vi "main.vi"() -> ()   [LabVIEW 2019]
uses:
  System.Speech
panel:
  in  "Tab Control":T1(tab)
  out "B out 2":bool[][](array[boolean])
  out "A+B 4":bool[][](array[boolean])
  out "A out 2":bool[][](array[boolean])
  in  "A in 2":dbl
  in  "B in 2":dbl
  out "A+B 3":dbl
  out "NUMBER  2":string
  in  "A in":dbl
  in  "B in":dbl
  out "A+B 2":dbl
  out "B out":bool[](array[boolean])
  out "A out":bool[](array[boolean])
  out "A+B":bool[][](array[boolean])
  out "NUMBER":string
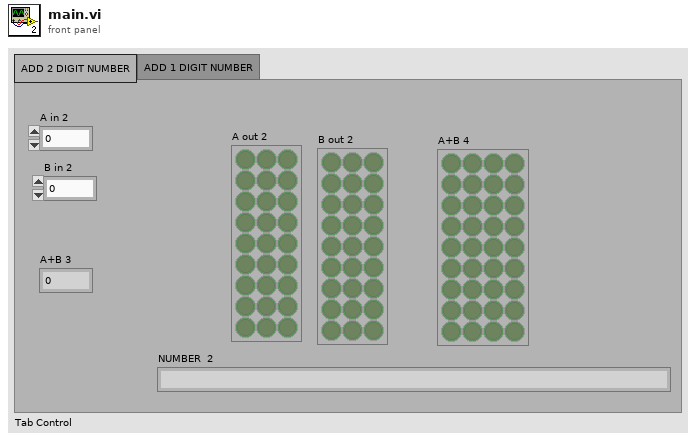
[diagram p1: front panel]
types:
  T1 = enum32{"ADD 2 DIGIT NUMBER", "ADD 1 DIGIT NUMBER"}
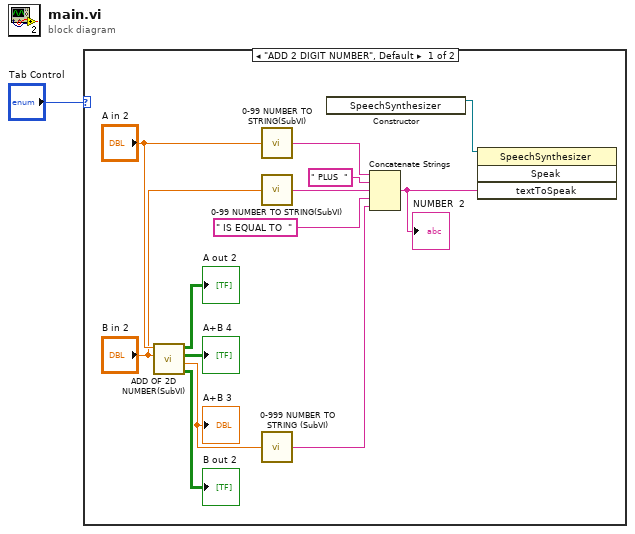
[diagram p0: block diagram]
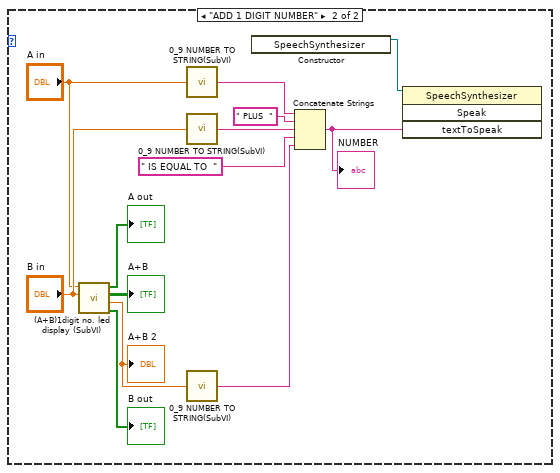
[diagram p2: hidden frame]
diagram:
  n1 = case shown="\"ADD 2 DIGIT NUMBER\", Default" "Tab Control" {
    frame "ADD 2 DIGIT NUMBER", Default {
      n2 = call "ADD OF 2D NUMBER(SubVI).vi"("B in"="B in 2", "A in"="A in 2") -> ("B out"=→"B out 2":bool[][], "A+B 2"=w2:dbl, "A+B"=→"A+B 4":bool[][], "A out"=→"A out 2":bool[][])  [unwired: 2 in]
      "A+B 3" <- w2
      n3 = call "0-99 NUMBER TO STRING(SubVI).vi"("A"="A in 2") -> ("element"=w9:string)
      n4 = call "0-99 NUMBER TO STRING(SubVI).vi"("A"="B in 2") -> ("element"=w7:string)
      n5 = call "0-999 NUMBER TO STRING (SubVI).vi"("A"=w2) -> ("element"=w3:string)
      n6 = constructor class="SpeechSynthesizer"() -> (reference out=w5:refnum<k24>)  [unwired: 3 in, 2 out]
      n7 = Concatenate Strings(w9, " PLUS  ", w7, " IS EQUAL TO  ", w3) -> (w4:string)
      "NUMBER  2" <- w4
      n8 = invoke class="SpeechSynthesizer" method="Speak"(reference=w5, "textToSpeak"=w4) -> ()  [unwired: 2 in, 4 out]
    }
    frame "ADD 1 DIGIT NUMBER" {
      n9 = call "(A+B)1digit no. led display (SubVI).vi"("B in"="B in", "A in"="A in") -> ("B out"=→"B out":bool[], "A+B 2"=w18:dbl, "A+B"=→"A+B":bool[][], "A out"=→"A out":bool[])  [unwired: 2 in]
      "A+B 2" <- w18
      n10 = call "0_9 NUMBER TO STRING(SubVI).vi"("A"="A in") -> ("element"=w22:string)
      n11 = call "0_9 NUMBER TO STRING(SubVI).vi"("A"="B in") -> ("element"=w20:string)
      n12 = call "0_9 NUMBER TO STRING(SubVI).vi"("A"=w18) -> ("element"=w17:string)
      n13 = constructor class="SpeechSynthesizer"() -> (reference out=w16:refnum<k24>)  [unwired: 3 in, 2 out]
      n14 = Concatenate Strings(w22, " PLUS  ", w20, " IS EQUAL TO  ", w17) -> (w15:string)
      "NUMBER" <- w15
      n15 = invoke class="SpeechSynthesizer" method="Speak"(reference=w16, "textToSpeak"=w15) -> ()  [unwired: 2 in, 4 out]
    }
  }
